vi "Actor Core.vi"(8 "error in":errorcluster, 11 "PointMotionView In":refnum<class "PointMotionView.lvclass">) -> (0 "error out":errorcluster, 3 "Actor out":refnum<class "Actor.lvclass">)   [LabVIEW 2020, in "PointMotionView.lvlib" / "PointMotionView.lvclass"]
uses:
  PointMotionView.lvclass
  C:/Program Files (x86)/National Instruments/LabVIEW 2020/vi.lib/gpm_packages/@cs/mva-viewable/Source/ActorEvents/IEventAggregator/IEventAggregator.lvclass
  <vilib>/ActorFramework/Actor/Actor.lvclass
  Controls/Axis_Control.ctl
  <vilib>/event_ctls.llb/lveventtype.ctl
  PointMotionView.lvclass/PointMotionView.ctl
  <vilib>/gpm_packages/@cs/mva-dialogbox/source/IDialogBox/IDialogBox/IDialogBox.lvclass
  <vilib>/gpm_packages/@cs/mva-viewable/Source/ActorEvents/IEventAggregator/IEventAggregator.lvclass
  Controls/Controls.lvlib
panel:
  in  "Start Run":bool
  in  "Axis":T1 caption="轴号"
  in  "smoothTime(Sec)":dbl caption="平滑时间(Sec)"
  in  "Deceleration(mm/Sec^2)":dbl caption="减速度(mm/Sec^2)"
  in  "Acceleration(mm/Sec^2)":dbl caption="加速度(mm/Sec^2)"
  in  "StepSize(mm)":dbl caption="步长(mm)"
  in  "velocity(mm/Sec)":dbl caption="速度(mm/Sec)"
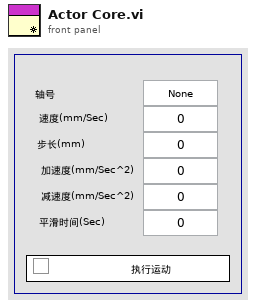
[diagram p1: front panel]
types:
  T1 = typedef "Controls.lvlib/Axis_Control.ctl" = enum16{"None", "1", "2", "3", "4", "5", "6", "7", "8"}
  T2 = typedef "lveventtype.ctl" = enum32{"Null", "Timeout", "Annotation Menu Selection", "Annotation Menu Selection?", "App Instance Close", "App Instance Close?", "Autoscale Range Change", "Bookmark Info Change", "Cell Edit", "Cell Edit?", "Cursor Grab", "Cursor Grab?", "Cursor Menu Selection", "Cursor Menu Selection?", "Cursor Move", "Cursor Release", "Data Change", "Direction Change", "Display State Change", "Drag Ended", "Drag Enter", "Drag Leave", "Drag Over", "Drag Source Update", "Drag Starting", "Drag Starting?", "Drop", "Exec State Change", "Key Down", "Key Down?", "Key Repeat", "Key Repeat?", "Key Up", "Listbox Double Click", "Menu Activation?", "Menu Selection (App)", "Menu Selection? (App)", "Menu Selection (User)", "Mouse Down", "Mouse Down?", "Mouse Enter", "Mouse Leave", "Mouse Move", "Mouse Up", "Mouse Wheel", "NI Security User Change (App)", "Pane Size", "Panel Close", "Panel Close?", "Panel Resize", "Plot Attribute Change", "Scale Range Change", "Shortcut Menu Activation?", "Shortcut Menu Selection (App)", "Shortcut Menu Selection? (App)", "Shortcut Menu Selection (User)", "Tree Double Click", "Tree Drag", "Tree Drag?", "Tree Drop", "Tree Drop?", "Tree Item Close", "Tree Item Close?", "Tree Item Open", "Tree Item Open?", "User Event", "Value Change"}
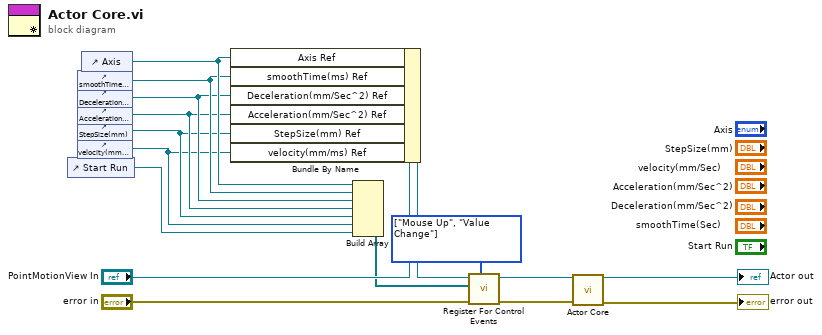
[diagram p0: block diagram]
diagram:
  w2 = T2[] [enum."Mouse Up", enum."Value Change"] items=["Null", "Timeout", "Annotation Menu Selection", "Annotation Menu Selection?", "App Instance Close", "App Instance Close?", "Autoscale Range Change", "Bookmark Info Change", "Cell Edit", "Cell Edit?", "Cursor Grab", "Cursor Grab?", "Cursor Menu Selection", "Cursor Menu Selection?", "Cursor Move", "Cursor Release", "Data Change", "Direction Change", "Display State Change", "Drag Ended", "Drag Enter", "Drag Leave", "Drag Over", "Drag Source Update", "Drag Starting", "Drag Starting?", "Drop", "Exec State Change", "Key Down", "Key Down?", "Key Repeat", "Key Repeat?", "Key Up", "Listbox Double Click", "Menu Activation?", "Menu Selection (App)", "Menu Selection? (App)", "Menu Selection (User)", "Mouse Down", "Mouse Down?", "Mouse Enter", "Mouse Leave", "Mouse Move", "Mouse Up", "Mouse Wheel", "NI Security User Change (App)", "Pane Size", "Panel Close", "Panel Close?", "Panel Resize", "Plot Attribute Change", "Scale Range Change", "Shortcut Menu Activation?", "Shortcut Menu Selection (App)", "Shortcut Menu Selection? (App)", "Shortcut Menu Selection (User)", "Tree Double Click", "Tree Drag", "Tree Drag?", "Tree Drop", "Tree Drop?", "Tree Item Close", "Tree Item Close?", "Tree Item Open", "Tree Item Open?", "User Event", "Value Change"] ("Registration Types")
  n1 = control-ref of="Start Run"() -> (w3:refnum<vi>)
  n2 = control-ref of="smoothTime(Sec)"() -> (w9:refnum<vi>)
  n3 = control-ref of="Deceleration(mm/Sec^2)"() -> (w8:refnum<vi>)
  n4 = control-ref of="Acceleration(mm/Sec^2)"() -> (w7:refnum<vi>)
  n5 = control-ref of="StepSize(mm)"() -> (w6:refnum<vi>)
  n6 = control-ref of="velocity(mm/Sec)"() -> (w5:refnum<vi>)
  n7 = control-ref of="Axis"() -> (w10:refnum<vi>)
  n8 = Bundle By Name(cluster="PointMotionView In", "Axis Ref"=w10, "smoothTime(ms) Ref"=w9, "Deceleration(mm/Sec^2) Ref"=w8, "Acceleration(mm/Sec^2) Ref"=w7, "StepSize(mm) Ref"=w6, "velocity(mm/ms) Ref"=w5) -> (w13:refnum<class "PointMotionView.lvclass">)
  n9 = Build Array(w10, w9, w8, w7, w6, w5, w3) -> (w4:refnum<vi>[])
  n10 = call <vilib>:"Register For Control Events.vi"("error in (no error)"="error in", "Registration Types"=w2, "Control Refnums"=w4, "IEventAggregator In"=w13) -> ("error out"=w11:errorcluster, "IEventAggregator Out"=w12:refnum<class "PointMotionView.lvclass">)  [unwired: 6 in]
  n11 = call-parent "Actor Core.vi"("error in"=w11, "IViewable In"=w12) -> ("error out"=→"error out":errorcluster, "Actor out"=→"Actor out":refnum<class "Actor.lvclass">)  [unwired: 8 in]
